vi "RTLSDR Global Variables.vi"() -> ()   [LabVIEW 2017]
panel:
  in  "Sample Rate":u32=2400000
  in  "Center Frequency":u32=100000000
  in  "RTLSDR Device Handle":u64
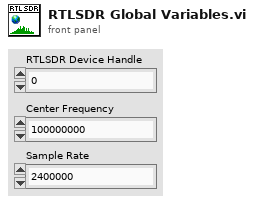
[diagram p1: front panel]
diagram:
